vi "지진 계측기 프로젝트2.vi"() -> ()   [LabVIEW 2021]
uses:
  <vilib>/Utility/sysdir.llb/System Directory Type.ctl
  <vilib>/numeric/Random Number (Range) U64.vi
panel:
  in  "정지":bool
  in  "파일저장":bool
  in  "알람리셋":bool
  in  "감지시작":bool
  out "알림":bool
  out "출력메시지":string
  out "지진센서값출력":dbl(graph)
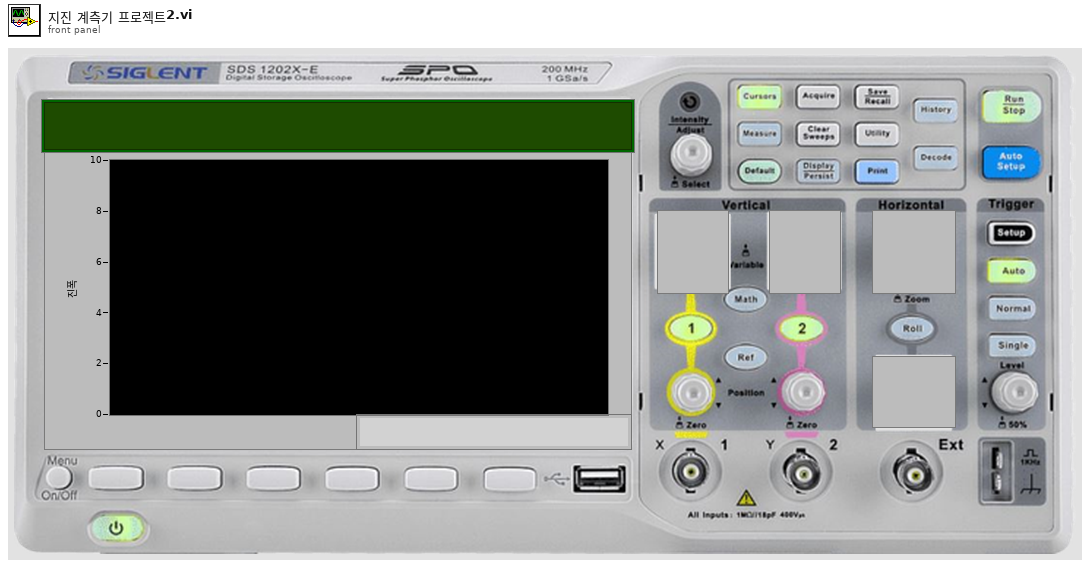
[diagram p1: front panel]
types:
  T1 = typedef "지진 계측기 상태 열거형 상수.ctl" = enum16{"초기화", "대기", "감지 시작", "알림 리셋", "정지"}
  T2 = cluster{"상태":T1, "알림":bool, "출력메시지":string, "지진센서값":dbl, "시간상수":i32}
  T3 = typedef "컨트롤 5.ctl" = enum16{"초기화", "대기", "감지시작", "알람리셋", "정지", "파일저장"}
  T4 = enum16{"open", "replace", "create", "open or create", "replace or create", "replace or create with confirmation"}
  T5 = typedef "System Directory Type.ctl" = i32
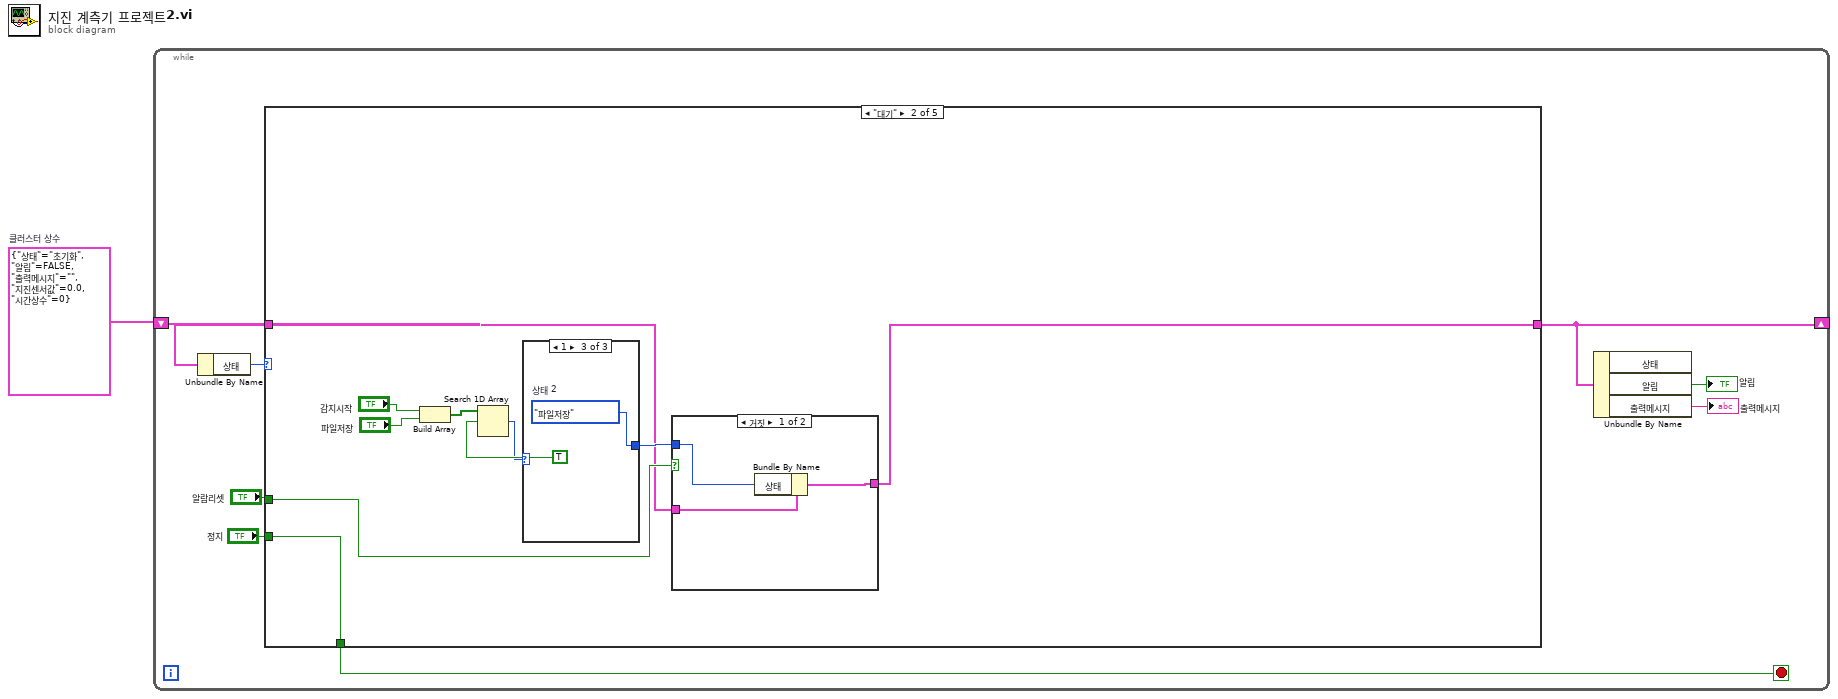
[diagram p0: block diagram]
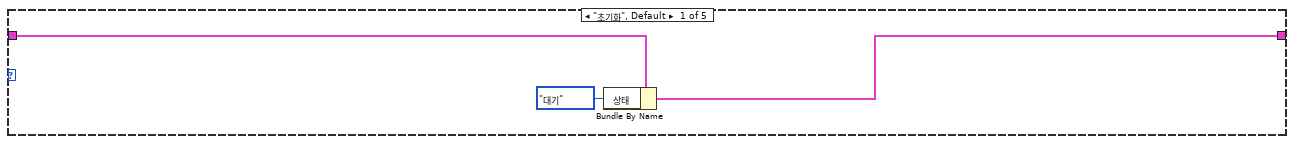
[diagram p2: hidden frame]
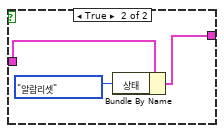
[diagram p3: hidden frame]
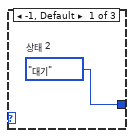
[diagram p4: hidden frame]
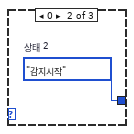
[diagram p5: hidden frame]
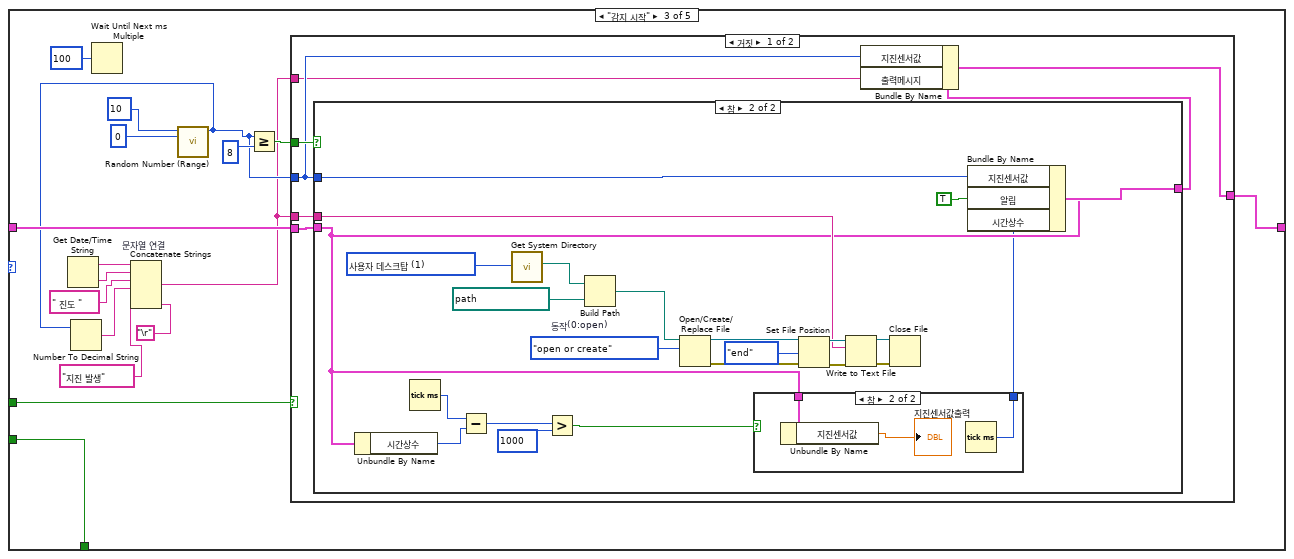
[diagram p6: hidden frame]
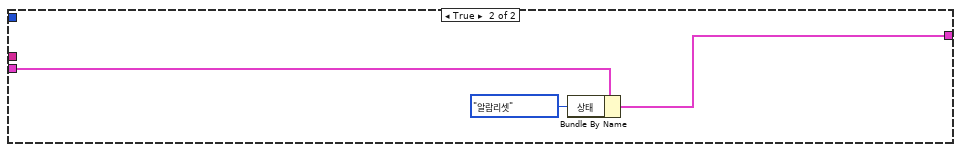
[diagram p9: hidden frame]
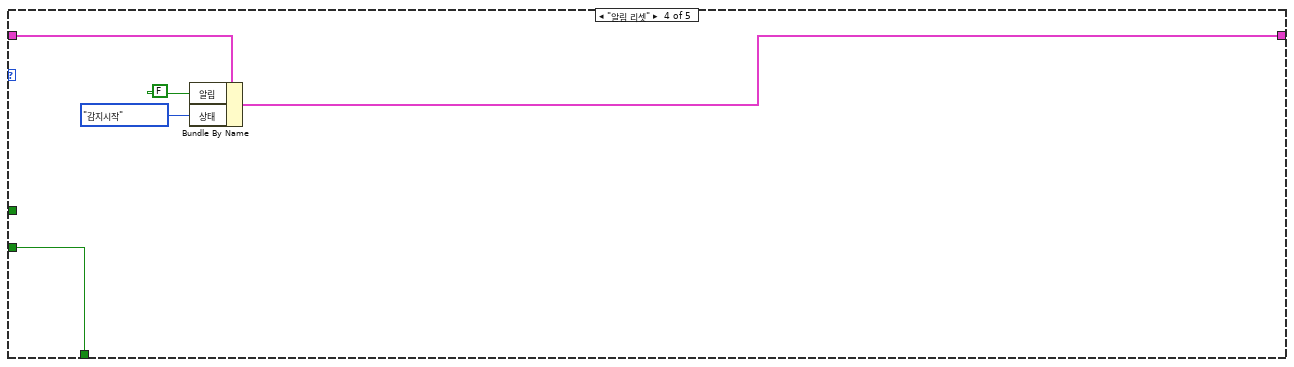
[diagram p10: hidden frame]
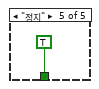
[diagram p11: hidden frame]
diagram:
  w1 = T2 {"상태"=enum."초기화", "알림"=FALSE, "출력메시지"="", "지진센서값"=0.0, "시간상수"=0}  # 클러스터 상수
  n1 = while {
    shift-right: [w8] -> _
    shift-left: w1 -> [w9]
    stop <- w7 stop-if-true
    n2 = Unbundle By Name(w9) -> ("상태"=w2:T1)
    n3 = case shown="\"대기\"" w2 {
      tunnel: [w11 w15 w43 w87 _] -> w8
      tunnel: w9 -> [w12 w13 w42 w90 _]
      tunnel: [_ w14 w32 w86 TRUE] -> w7
      tunnel: "알람리셋" -> [_ w17 w41 _ _]
      tunnel: "정지" -> [_ w14 w32 w86 _]
      frame "초기화", Default {
        n4 = Bundle By Name(cluster=w12, "상태"=지진_계측기_상태_열거형_상수."대기") -> (w11:T2)
      }
      frame "대기" {
        n5 = Build Array("감지시작", "파일저장") -> (w22:bool[])
        n6 = Search 1D Array(1D array=w22, element=TRUE ("원소")) -> (index of element=w20:i32)  [unwired: 1 in]
        n7 = case shown="1" w20 {
          tunnel: [w29 w30 w31] -> w16
          frame -1, Default {
            w29 = 지진_계측기_상태_열거형_상수."대기"  # 상태 2
          }
          frame 0 {
            w30 = 컨트롤_5."감지시작"  # 상태 2
          }
          frame 1 {
            w31 = 컨트롤_5."파일저장"  # 상태 2
          }
        }
        n8 = case shown="거짓" w17 {
          tunnel: w16 -> [w23 _]
          tunnel: [w24 w28] -> w15
          tunnel: w13 -> [w25 w27]
          frame False {
            n9 = Bundle By Name(cluster=w25, "상태"=w23) -> (w24:T2)
          }
          frame True {
            n10 = Bundle By Name(cluster=w27, "상태"=컨트롤_5."알람리셋") -> (w28:T2)
          }
        }
      }
      frame "감지 시작" {
        n11 = Get Date/Time String() -> (date string=w37:string, time string=w36:string)  [unwired: 3 in]
        n12 = Wait Until Next ms Multiple(millisecond multiple=u32 100 ("ms 배수")) -> ()  [unwired: 1 out]
        n13 = call-poly <vilib>:"Random Number (Range).vi"("lower bound (0)"=u64 0, "upper bound (100)"=u64 10) -> ("number"=w34:u64)  [unwired: 9 in]
        n14 = Number To Decimal String(number=w34) -> (decimal integer string=w35:string)  [unwired: 1 in]
        n15 = Concatenate Strings "문자열 연결"(w37, w36, " 진도 " ("문자열"), w35, "지진 발생" ("문자열"), "\r") -> (w33:string)
        n16 = Greater Or Equal?(x=w34, y=u64 8) -> (x >= y?=w44:bool)
        n17 = case shown="거짓" w41 {
          tunnel: w44 -> [w55 _]
          tunnel: [w53 w84] -> w43
          tunnel: w42 -> [w52 w85]
          tunnel: w34 -> [w51 _]
          tunnel: w33 -> [w50 _]
          tunnel: w33 -> [w49 _]
          frame False {
            n18 = case shown="참" w55 {
              tunnel: w52 -> [w56 w58]
              tunnel: w51 -> [_ w79]
              tunnel: [w56 w78] -> w54
              tunnel: w49 -> [_ w65]
              frame False {
              }
              frame True {
                w68 = T4."open or create"  # 동작(0:open)
                w66 = T5 1 items=["사용자 홈"=0, "사용자 데스크탑"=1, "사용자 문서"=2, "사용자 어플리케이션 데이터"=3, "사용자 환경"=4, "사용자 임시"=5, "퍼블릭 문서"=6, "퍼블릭 어플리케이션 데이터"=7, "퍼블릭 환경"=8, "퍼블릭 캐시"=13, "시스템 코어 라이브러리"=9, "시스템 설치된 라이브러리"=10, "어플리케이션 파일"=11, "부팅 볼륨 루트"=12] ("system directory type")
                n19 = Unbundle By Name(w58) -> ("시간상수"=w62:i32)
                n20 = Tick Count (ms)() -> (millisecond timer value=w63:u32)
                n21 = Subtract(x=w63, y=w62) -> (x-y=w61:u32)
                n22 = call <vilib>:"Get System Directory.vi"("system directory type"=w66) -> ("system directory"=w64:path)  [unwired: 10 in]
                n23 = Greater?(x=w61, y=u32 1000) -> (0:w59:bool)
                n24 = Build Path ("경로 만들기")(base path=w64, name or relative path=path "날짜_Log.txt" ("이름 또는 상대 경로")) -> (appended path=w76:path)
                n25 = Open/Create/Replace File ("파일 열기/생성/대체")(file path (use dialog)=w76, operation (0:open)=w68) -> (refnum out=w71:refnum<file>, error out=w70:errorcluster)  [unwired: 4 in, 1 out]
                n26 = case shown="참" w59 {
                  tunnel: w58 -> [_ w82]
                  tunnel: [_ w80] -> w57
                  frame False {
                  }
                  frame True {
                    n27 = Unbundle By Name(w82) -> ("지진센서값"=→"지진센서값출력":dbl)
                    n28 = Tick Count (ms)() -> (millisecond timer value=w80:u32)
                  }
                }
                n29 = Set File Position ("파일 위치 설정")(refnum=w71, from (0:start)=enum16{"start", "end", "current"}."end" ("위치(0:start)"), error in=w70) -> (refnum out=w73:refnum<file>, error out=w72:errorcluster)  [unwired: 1 in]
                n30 = Write to Text File ("텍스트 파일에 쓰기")(file (use dialog)=w73, text=w65, error in=w72) -> (refnum out=w75:refnum<file>, error out=w74:errorcluster)  [unwired: 1 in, 1 out]
                n31 = Close File ("파일 닫기")(refnum=w75, error in=w74) -> ()  [unwired: 2 out]
                n32 = Bundle By Name(cluster=w58, "지진센서값"=w79, "알림"=TRUE, "시간상수"=w57) -> (w78:T2)
              }
            }
            n33 = Bundle By Name(cluster=w54, "지진센서값"=w51, "출력메시지"=w50) -> (w53:T2)
          }
          frame True {
            n34 = Bundle By Name(cluster=w85, "상태"=컨트롤_5."알람리셋") -> (w84:T2)
          }
        }
      }
      frame "알림 리셋" {
        n35 = Bundle By Name(cluster=w90, "알림"=FALSE, "상태"=컨트롤_5."감지시작") -> (w87:T2)
      }
      frame "정지" {
      }
    }
    n36 = Unbundle By Name(w8) -> ("알림"=→"알림":bool, "출력메시지"=→"출력메시지":string)  [unwired: 1 out]
  }
